vi "find_best_match.vi"(7 "radius":dbl=5.0, 8 "error in (no error)":errorcluster, 10 "location (x/y/z)":dbl[](array[numeric]), 11 "PointCollection in":refnum<class "PointCollection.lvclass">) -> (0 "error out":errorcluster, 1 "found?":bool, 2 "point (x/y/z)":dbl[](array[numeric]), 3 "PointCollection out":refnum<class "PointCollection.lvclass">)   [LabVIEW 2010, in "PointCollection.lvclass"]
uses:
  PointCollection.lvclass
  mode_enum.ctl
panel:
  out "distance":dbl
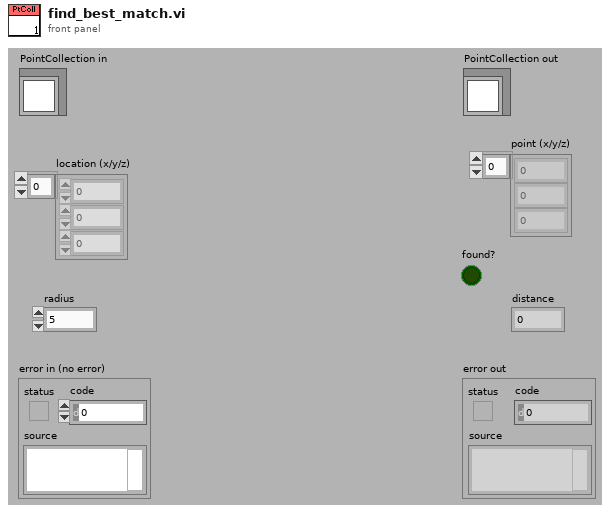
[diagram p1: front panel]
types:
  T1 = typedef "PointCollection.lvclass/mode_enum.ctl" = enum16{"points first", "dimensions first"}
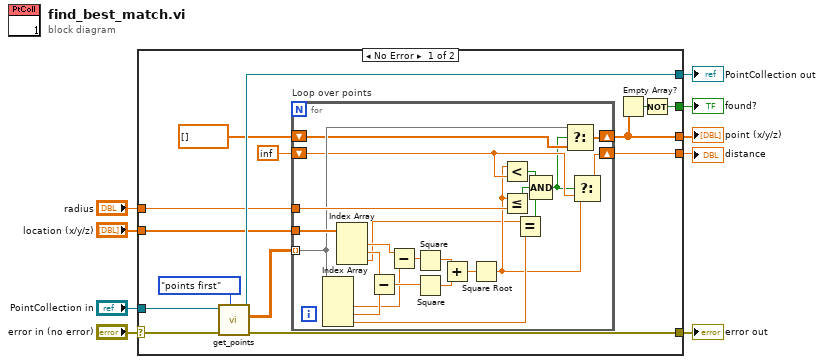
[diagram p0: block diagram]
diagram:
  n1 = case shown="No Error" "error in (no error)" {
    selector: "error in (no error)" -> [w23 w48]
    tunnel: [w13 w48] -> w8
    tunnel: [w21 w47] -> w6
    tunnel: "PointCollection in" -> [w22 w47]
    tunnel: "location (x/y/z)" -> [w18 _]
    tunnel: "radius" -> [w17 _]
    tunnel: [w11 _] -> w3
    tunnel: [w14 _] -> w2
    tunnel: [w10 _] -> w1
    frame No Error {
      n2 = call-dynamic "get_points.vi"("retrieval mode"=mode_enum."points first", "error in (no error)"=w23, "PointCollection in"=w22) -> ("error out"=w13:errorcluster, "points"=w20:dbl[][], "PointCollection out"=w21:refnum<class "PointCollection.lvclass">)  [unwired: 6 in]
      n3 = for "Loop over points" {
        tunnel: w20 -> [w39] mode=indexing
        tunnel: w18 -> [w46]
        tunnel: w17 -> [w40]
        shift-right: [w38] -> w11
        shift-left: dbl[] [] ("points") -> [w36]
        shift-right: [w37] -> w10
        shift-left: inf -> [w35]
        n4 = Index Array(array=w39) -> (element #2=w32:dbl, element #3=w33:dbl, element #4=w34:dbl)  [unwired: 4 in, 1 out]
        n5 = Index Array(array=w46) -> (element #1=w26:dbl, element #2=w25:dbl, element #3=w24:dbl)  [unwired: 3 in]
        n6 = Subtract(x=w25, y=w33) -> (x-y=w44:dbl)
        n7 = Subtract(x=w26, y=w32) -> (x-y=w45:dbl)
        n8 = Square(x=w45) -> (x^2=w43:dbl)
        n9 = Square(x=w44) -> (x^2=w42:dbl)
        n10 = Add(x=w43, y=w42) -> (x+y=w41:dbl)
        n11 = Square Root(x=w41) -> (sqrt(x)=w27:dbl)
        n12 = Less?(x=w27, y=w35) -> (x < y?=w30:bool)
        n13 = Less Or Equal?(x=w27, y=w40) -> (x <= y?=w28:bool)
        n14 = Equal?(x=w24, y=w34) -> (x = y?=w31:bool)
        n15 = Compound Arithmetic op=AND(w30, w28, w31) -> (w29:bool)
        n16 = Select(t=w39, s=w29, f=w36) -> (s? t:f=w38:dbl[])
        n17 = Select(t=w27, s=w29, f=w35) -> (s? t:f=w37:dbl)
      }
      n18 = Empty Array?(array=w11) -> (empty?=w15:bool)
      n19 = Not(x=w15) -> (.not. x?=w14:bool)
    }
    frame Error {
    }
  }
  "error out" <- w8
  "PointCollection out" <- w6
  "point (x/y/z)" <- w3
  "found?" <- w2
  "distance" <- w1
